vi "PSCOMMON_All Modules Queue.vi"() -> (2 "All Queues":T1)   [LabVIEW 2016]
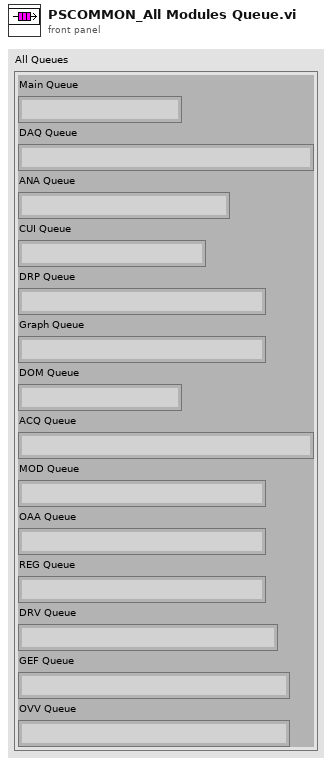
[diagram p1: front panel]
types:
  T1 = cluster{"Main Queue":string, "DAQ Queue":string, "ANA Queue":string, "CUI Queue":string, "DRP Queue":string, "Graph Queue":string, "DOM Queue":string, "ACQ Queue":string, "MOD Queue":string, "OAA Queue":string, "REG Queue":string, "DRV Queue":string, "GEF Queue":string, "OVV Queue":string}
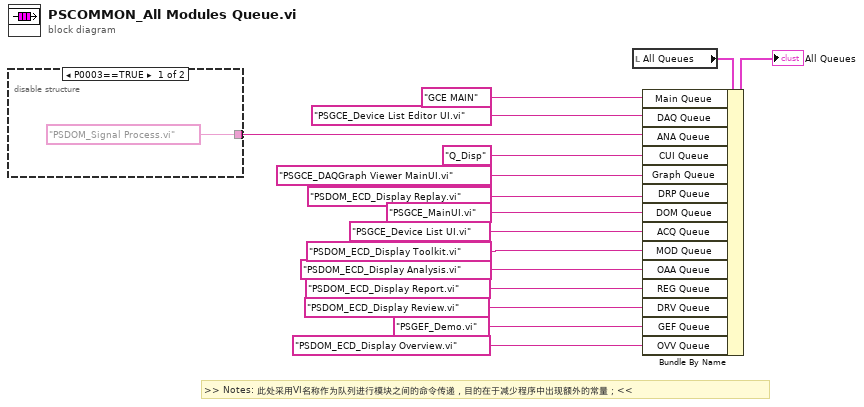
[diagram p0: block diagram]
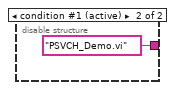
[diagram p2: hidden frame]
diagram:
  # ">> Notes: 此处采用VI名称作为队列进行模块之间的命令传递，目的在于减少程序中出现额外的常量；<<"
  n1 = disable-structure shown="P0003==TRUE" {
    disable-tunnel: ["PSDOM_Signal Process.vi" ("Name") "PSVCH_Demo.vi" ("Name")] -> w9
    frame condition #0 {
    }
    frame condition #1 (active) {
    }
  }
  n2 = local read "All Queues"() -> (w12:T1)
  n3 = Bundle By Name(cluster=w12, "Main Queue"="GCE MAIN", "DAQ Queue"="PSGCE_Device List Editor UI.vi" ("Name"), "ANA Queue"=w9, "CUI Queue"="Q_Disp" ("QueueName"), "Graph Queue"="PSGCE_DAQGraph Viewer MainUI.vi" ("Name"), "DRP Queue"="PSDOM_ECD_Display Replay.vi" ("QueueName"), "DOM Queue"="PSGCE_MainUI.vi" ("Name"), "ACQ Queue"="PSGCE_Device List UI.vi" ("Name"), "MOD Queue"="PSDOM_ECD_Display Toolkit.vi" ("Name"), "OAA Queue"="PSDOM_ECD_Display Analysis.vi" ("Name"), "REG Queue"="PSDOM_ECD_Display Report.vi" ("Name"), "DRV Queue"="PSDOM_ECD_Display Review.vi" ("Name"), "GEF Queue"="PSGEF_Demo.vi" ("Name"), "OVV Queue"="PSDOM_ECD_Display Overview.vi" ("Name")) -> (→"All Queues":T1)
